vi "VNA - Initiate and Fetch - Dual Port.vi"(0 "Semiconductor Module Context":T1, 5 "VNA Calibration Parameters":T2, 11 "error in (no error)":errorcluster) -> (6 "Instrument Sessions Out":refnum<k15>[](array[refnum]), 13 "Port 1 Capacitance":dbl[](array[numeric]), 14 "Port 2 Capacitance":dbl[](array[numeric]), 15 "error out":errorcluster)   [LabVIEW 2013]
doc: "Initiates and fetches niVNA S11 measurements and converts it to a capacitance measurement."
uses:
  VNA Calibration Parameters.ctl
  <vilib>/NI_TestStand_SemiconductorModule/NI_TestStand_Semiconductor_Module.lvlibp/PinMap/General/SemiconductorModuleContext.ctl
  <instrlib>/niVNA/niVNA.llb/niVNA Fetch Receiver Measurement Complex (CDB).vi
  Pin Map API/VNA Custom Instrument.lvlib
  <vilib>/NI_TestStand_SemiconductorModule/NI_TestStand_Semiconductor_Module.lvlibp
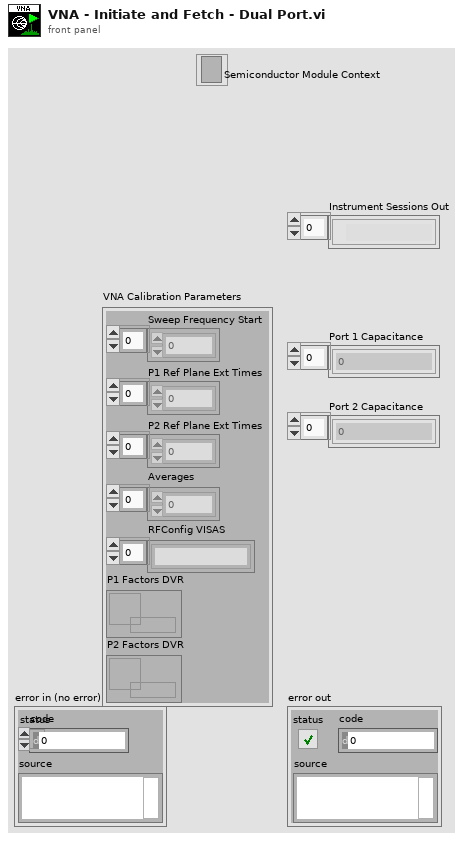
[diagram p1: front panel]
types:
  T1 = typedef "NI_TestStand_Semiconductor_Module.lvlibp/SemiconductorModuleContext.ctl" = refnum<k7>
  T2 = typedef "VNA Calibration Parameters.ctl" = cluster{"Sweep Frequency Start":dbl[], "P1 Ref Plane Ext Times":dbl[], "P2 Ref Plane Ext Times":dbl[], "Averages":i32[], "RFConfig VISAS":string[], "P1 Factors DVR":refnum<data-value>, "P2 Factors DVR":refnum<data-value>}
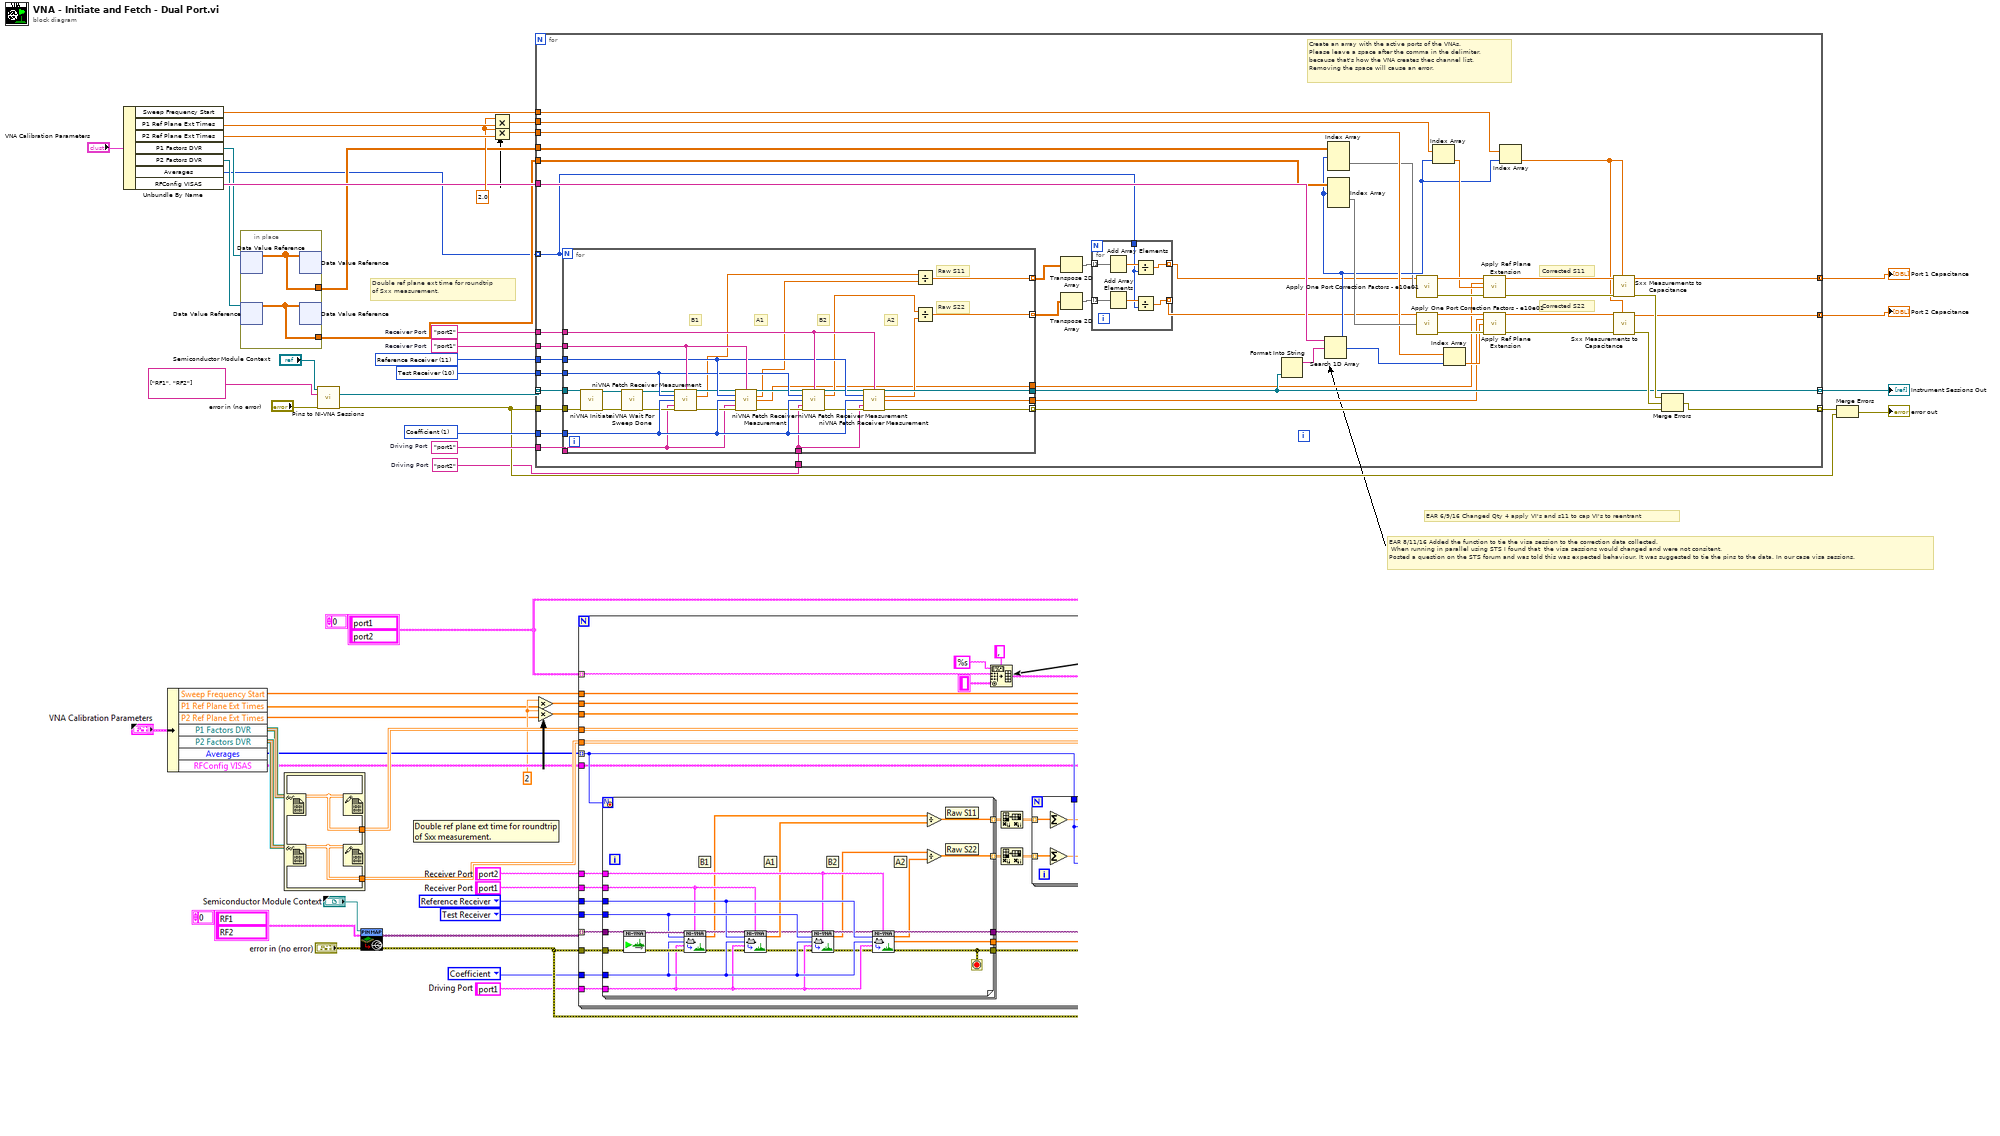
[diagram p0: block diagram]
diagram:
  w4 = "port2"  # Driving Port
  w16 = 1 items=["Impedance", "Coefficient"] ("format")
  w22 = "port2"  # Receiver Port
  w19 = 10 items=["Test Receiver"=10, "Reference Receiver"=11] ("receiver")
  w18 = "port1"  # Driving Port
  w21 = "port1"  # Receiver Port
  w20 = 11 items=["Test Receiver"=10, "Reference Receiver"=11] ("receiver")
  w23 = 2.0
  # "EAR 8/11/16 Added the function to tie the visa session to the correction data collected.\n When running in parallel using STS I found that  the visa sessions would changed and were not consitent. \nPosted a question on the STS forum and was told this was expected behaviour. It was suggested to tie the pins to the data. In our case visa sessions."
  # "EAR 6/9/16 Changed Qty 4 apply VI's and s11 to cap VI's to reentrant"
  # "Double ref plane ext time for roundtrip\nof Sxx measurement."
  n1 = Unbundle By Name("VNA Calibration Parameters") -> ("Sweep Frequency Start"=w17:dbl[], "P1 Ref Plane Ext Times"=w24:dbl[], "P2 Ref Plane Ext Times"=w25:dbl[], "P1 Factors DVR"=w7:refnum<data-value>, "P2 Factors DVR"=w5:refnum<data-value>, "Averages"=w1:i32[], "RFConfig VISAS"=w15:string[])
  n2 = in-place {
    in-place-border: [w31] -> w8
    in-place-border: [w32] -> w6
    n3 = in-place-dvr #1(w7) -> (w31:cdb[][][])  [unwired: 1 out]
    n4 = in-place-dvr #2(w5) -> (w32:cdb[][][])  [unwired: 1 out]
    n5 = in-place-dvr #1(w31) -> ()  [unwired: 2 out]
    n6 = in-place-dvr #2(w32) -> ()  [unwired: 2 out]
  }
  n7 = call "Pins to NI-VNA Sessions.vi"("Semiconductor Module Context"="Semiconductor Module Context", "Pins"=string[] ["RF1", "RF2"], "error in (no error)"="error in (no error)") -> ("Instrument Sessions"=w11:refnum<k15>[], "error out"=w10:errorcluster)  [unwired: 8 in, 3 out]
  n8 = Multiply(x=w23, y=w24) -> (x*y=w27:dbl[])
  n9 = Multiply(x=w23, y=w25) -> (x*y=w26:dbl[])
  n10 = for {
    tunnel: w10 -> [w78]
    tunnel: w11 -> [w77] mode=indexing
    tunnel: [w73] -> w28 mode=indexing
    tunnel: [w57] -> w29 mode=indexing
    tunnel: w6 -> [w53]
    tunnel: w8 -> [w54]
    tunnel: [w59] -> w3 mode=concatenating
    tunnel: [w58] -> w2 mode=concatenating
    tunnel: w27 -> [w51]
    tunnel: w26 -> [w49]
    tunnel: w22 -> [w64]
    tunnel: w21 -> [w63]
    tunnel: w20 -> [w62]
    tunnel: w19 -> [w61]
    tunnel: w16 -> [w60]
    tunnel: w18 -> [w44]
    tunnel: w17 -> [w46]
    tunnel: w15 -> [w56]
    tunnel: w4 -> [w43]
    tunnel: w1 -> [w33] mode=indexing
    # "Create an array with the active ports of the VNAs.\nPlease leave a space after the comma in the delimiter, \nbecause that's how the VNA creates thec channel list. \nRemoving the space will cause an error."
    # "Corrected S22"
    # "Corrected S11"
    n11 = for {
      N: w33 -> [_]
      tunnel: w78 -> [w114]
      tunnel: w77 -> [w113]
      tunnel: [w112] -> w74 mode=indexing
      tunnel: w64 -> [w111]
      tunnel: w63 -> [w110]
      tunnel: w62 -> [w109]
      tunnel: w61 -> [w108]
      tunnel: w60 -> [w107]
      tunnel: [w106] -> w57
      tunnel: [w95] -> w37 mode=indexing
      tunnel: [w94] -> w35 mode=indexing
      tunnel: w44 -> [w93]
      tunnel: w43 -> [w92]
      tunnel: [w87] -> w41
      tunnel: [w86] -> w40
      # "Raw S22"
      # "Raw S11"
      # "A2"
      # "B2"
      # "B1"
      # "A1"
      n12 = call <instrlib>:"niVNA Initiate.vi"("instrument handle"=w113, "error in"=w114) -> ("instrument handle out"=w99:refnum<k15>, "error out"=w98:errorcluster)  [unwired: 12 in]
      n13 = call <instrlib>:"niVNA Wait For Sweep Done.vi"("instrument handle"=w99, "error in"=w98) -> ("instrument handle out"=w97:refnum<k15>, "error out"=w96:errorcluster)  [unwired: 12 in]
      n14 = call-poly <instrlib>:"niVNA Fetch Receiver Measurement.vi"("instrument handle"=w97, "receiver port"=w110, "receiver"=w108, "format"=w107, "driving port"=w93, "error in"=w96) -> ("instrument handle out"=w101:refnum<k15>, "data"=w89:cdb[], "error out"=w100:errorcluster)  [unwired: 6 in, 1 out]
      n15 = call-poly <instrlib>:"niVNA Fetch Receiver Measurement.vi"("instrument handle"=w101, "receiver port"=w110, "receiver"=w109, "format"=w107, "driving port"=w93, "error in"=w100) -> ("instrument handle out"=w104:refnum<k15>, "data"=w90:cdb[], "scale points"=w87:dbl[], "error out"=w105:errorcluster)  [unwired: 6 in]
      n16 = call-poly <instrlib>:"niVNA Fetch Receiver Measurement.vi"("instrument handle"=w104, "receiver port"=w111, "receiver"=w108, "format"=w107, "driving port"=w92, "error in"=w105) -> ("instrument handle out"=w102:refnum<k15>, "data"=w91:cdb[], "error out"=w103:errorcluster)  [unwired: 6 in, 1 out]
      n17 = call-poly <instrlib>:"niVNA Fetch Receiver Measurement.vi"("instrument handle"=w102, "receiver port"=w111, "receiver"=w109, "format"=w107, "driving port"=w92, "error in"=w103) -> ("instrument handle out"=w106:refnum<k15>, "data"=w88:cdb[], "scale points"=w86:dbl[], "error out"=w112:errorcluster)  [unwired: 6 in]
      n18 = Divide(x=w89, y=w90) -> (x/y=w95:cdb[])
      n19 = Divide(x=w91, y=w88) -> (x/y=w94:cdb[])
    }
    n20 = Transpose 2D Array(2D array=w37) -> (transposed array=w39:cdb[][])
    n21 = Transpose 2D Array(2D array=w35) -> (transposed array=w38:cdb[][])
    n22 = for {
      tunnel: w39 -> [w85] mode=indexing
      tunnel: w38 -> [w84] mode=indexing
      tunnel: w33 -> [w81]
      tunnel: [w80] -> w36 mode=indexing
      tunnel: [w79] -> w34 mode=indexing
      n23 = Add Array Elements(numeric array=w85) -> (sum=w83:cdb)
      n24 = Add Array Elements(numeric array=w84) -> (sum=w82:cdb)
      n25 = Divide(x=w83, y=w81) -> (x/y=w80:cdb)
      n26 = Divide(x=w82, y=w81) -> (x/y=w79:cdb)
    }
    n27 = Format Into String(w57) -> (resulting string=w55:string)  [unwired: 3 in, 1 out]
    n28 = Search 1D Array(1D array=w56, element=w55) -> (index of element=w47:i32)  [unwired: 1 in]
    n29 = Index Array(array=w54, index (dim 0)=w47) -> (element=w42:cdb[][])  [unwired: 2 in]
    n30 = Index Array(array=w53, index (dim 0)=w47) -> (element=w52:cdb[][])  [unwired: 2 in]
    n31 = call "Apply One Port Correction Factors - e10e01.vi"("Raw Sxx Data"=w36, "One Port Correction Factors"=w42) -> ("Corrected Sxx Data"=w72:cdb[], "Error Out"=w69:errorcluster)  [unwired: 12 in]
    n32 = call "Apply One Port Correction Factors - e10e01.vi"("Raw Sxx Data"=w34, "One Port Correction Factors"=w52) -> ("Corrected Sxx Data"=w68:cdb[], "Error Out"=w67:errorcluster)  [unwired: 12 in]
    n33 = Index Array(array=w51, index=w47) -> (element=w50:dbl)
    n34 = Index Array(array=w49, index=w47) -> (element=w48:dbl)
    n35 = call "Apply Ref Plane Extension.vi"("Sxx Data"=w72, "Frequencies"=w41, "Ref Plane Extension Time"=w50, "Error In"=w69) -> ("Sxx Data - Ref Plane Shifted"=w71:cdb[], "Error Out"=w70:errorcluster)  [unwired: 10 in]
    n36 = call "Apply Ref Plane Extension.vi"("Sxx Data"=w68, "Frequencies"=w40, "Ref Plane Extension Time"=w48, "Error In"=w67) -> ("Sxx Data - Ref Plane Shifted"=w66:cdb[], "Error Out"=w65:errorcluster)  [unwired: 10 in]
    n37 = Index Array(array=w46, index=w47) -> (element=w45:dbl)
    n38 = call "Sxx Measurements to Capacitance.vi"("Sweep Frequency Start"=w45, "error in (no error)"=w70, "S11 Data"=w71) -> ("error out"=w76:errorcluster, "Capacitance"=w59:dbl[])  [unwired: 7 in]
    n39 = call "Sxx Measurements to Capacitance.vi"("Sweep Frequency Start"=w45, "error in (no error)"=w65, "S11 Data"=w66) -> ("error out"=w75:errorcluster, "Capacitance"=w58:dbl[])  [unwired: 7 in]
    n40 = Merge Errors(w76, w75, w74) -> (w73:errorcluster)
  }
  "Port 1 Capacitance" <- w3
  "Instrument Sessions Out" <- w29
  "Port 2 Capacitance" <- w2
  n41 = Merge Errors(w28, w10) -> (→"error out":errorcluster)
